vi "Name_Last Start Time.vi"() -> (3 "Name":string)   [LabVIEW 2015, in "Exposure Process.lvlib"]
uses:
  Exposure Process.lvlib
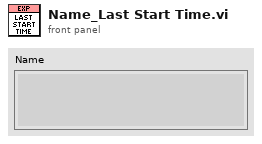
[diagram p1: front panel]
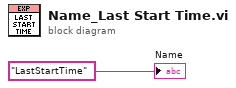
[diagram p0: block diagram]
diagram:
  "Name" <- "LastStartTime"
